vi "Room-Temperature Sensor Data.vi"(8 "error in (no error)":errorcluster, 11 "VISA resource name":refnum<visa-resource-name>) -> (0 "error out":errorcluster, 2 "Room-Temperature Sensor Data":dbl format="%.3f", 3 "VISA resource name out":refnum<visa-resource-name>)   [LabVIEW 2019, in "Lake Shore 325.lvlib"]
doc: "This VI returns the temperature reading in Kelvin measured by the built-in room-temperature compensation sensor."
uses:
  Lake Shore 325.lvlib
  Instance           1 36Saved   Room-Temperature Sensor Data .vi
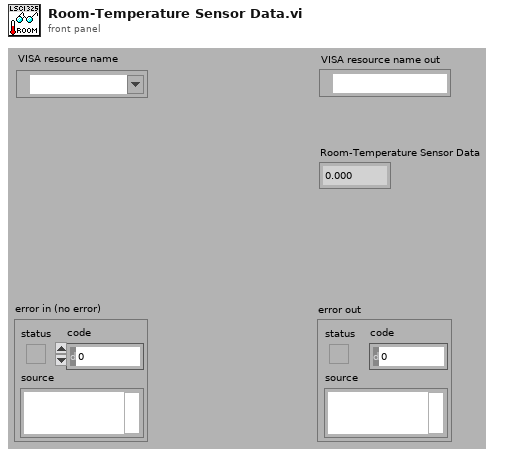
[diagram p1: front panel]
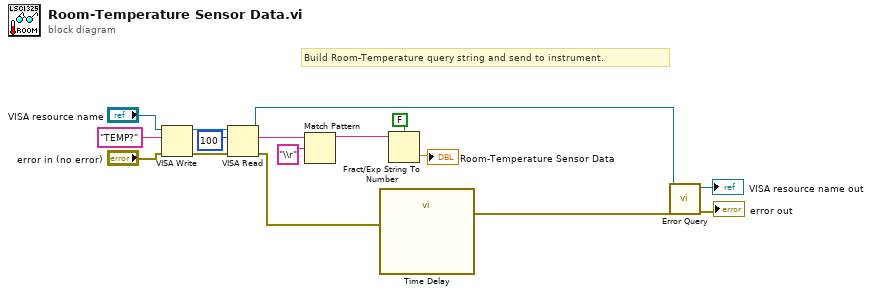
[diagram p0: block diagram]
diagram:
  # "Build Room-Temperature query string and send to instrument."
  n1 = VISA Write(VISA resource name="VISA resource name", write buffer="TEMP?", error in (no error)="error in (no error)") -> (VISA resource name out=w9:refnum<visa-resource-name>, error out=w8:errorcluster)  [unwired: 1 out]
  n2 = VISA Read(VISA resource name=w9, byte count=100, error in (no error)=w8) -> (VISA resource name out=w12:refnum<visa-resource-name>, read buffer=w11:string, error out=w2:errorcluster)  [unwired: 1 out]
  n3 = Match Pattern(string=w11, regular expression="\\r") -> (before substring=w5:string)  [unwired: 1 in, 3 out]
  n4 = call "Time Delay"("error in (no error)"=w2) -> ("error out"=w1:errorcluster)  [unwired: 10 in]
  n5 = Fract/Exp String To Number(use system decimal point (T)=FALSE, string=w5) -> (number=→"Room-Temperature Sensor Data":dbl)  [unwired: 2 in, 1 out]
  n6 = call "Error Query.vi"("error in (no error)"=w1, "VISA resource name"=w12) -> ("error out"=→"error out":errorcluster, "VISA resource name out"=→"VISA resource name out":refnum<visa-resource-name>)  [unwired: 7 in, 1 out]
